vi "1L11-tb1D_extraire_elements_de_liste_ch_selon_critere_n0.vi"(9 "critère":string, 10 "Liste valeurs":string[](array[string]), 11 "liste de chaîne":string[](array[string])) -> (3 "valeurs associées à critère":string[](array[string]))   [LabVIEW 2010, in "lv_01.lvlib"]
doc: "Soit 2 listes (tableau 1D) associées (Chaîne et Valeurs) : l'entrée [critère] est recherchée dans la liste des chaînes et le VI retourne toutes les valeurs associées au critère."
uses:
  lv_01.lvlib
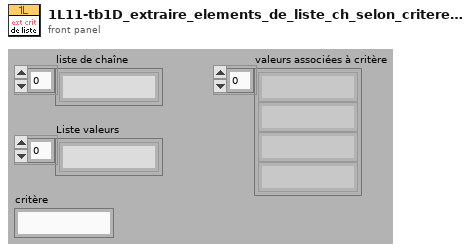
[diagram p1: front panel]
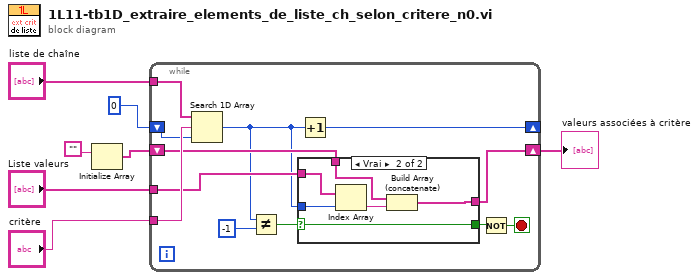
[diagram p0: block diagram]
diagram:
  n1 = Initialize Array("") -> (w5:string[])  [unwired: 1 in]
  n2 = while {
    tunnel: "liste de chaîne" -> [w19]
    tunnel: "critère" -> [w18]
    shift-right: [w17] -> _
    shift-left: 0 -> [w16]
    tunnel: "Liste valeurs" -> [w15]
    shift-right: [w12] -> w4
    shift-left: w5 -> [w11]
    stop <- w8 stop-if-true
    n3 = Search 1D Array(1D array=w19, element=w18, start index (0)=w16) -> (index of element=w10:i32)
    n4 = Not Equal?(x=w10, y=-1) -> (x != y?=w14:bool)
    n5 = case shown="Vrai" w14 {
      selector: w14 -> [w20 w22]
      tunnel: w15 -> [_ w25]
      tunnel: w10 -> [_ w24]
      tunnel: [w21 w27] -> w12
      tunnel: w11 -> [w21 w26]
      tunnel: [w20 w22] -> w9
      frame False {
      }
      frame True {
        n6 = Index Array(array=w25, index=w24) -> (element=w23:string)
        n7 = Build Array (concatenate)(w26, w23) -> (w27:string[])
      }
    }
    n8 = Increment(x=w10) -> (x+1=w17:i32)
    n9 = Not(x=w9) -> (.not. x?=w8:bool)
  }
  "valeurs associées à critère" <- w4
